vi "读写字节数组DEMO.vi"() -> ()   [LabVIEW 2012]
panel:
  out "Receive":dbl(graph)
  out "Send":dbl(graph)
  in  "停止":bool
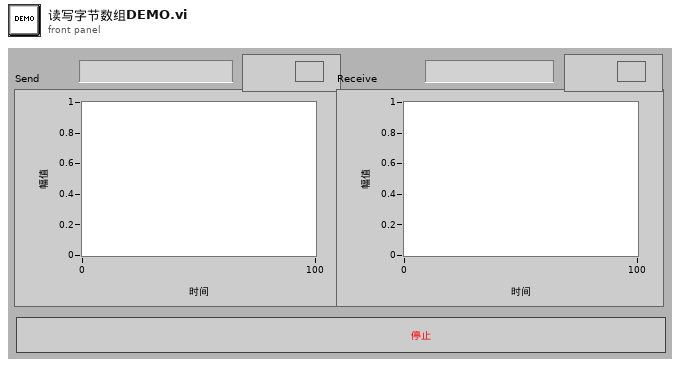
[diagram p1: front panel]
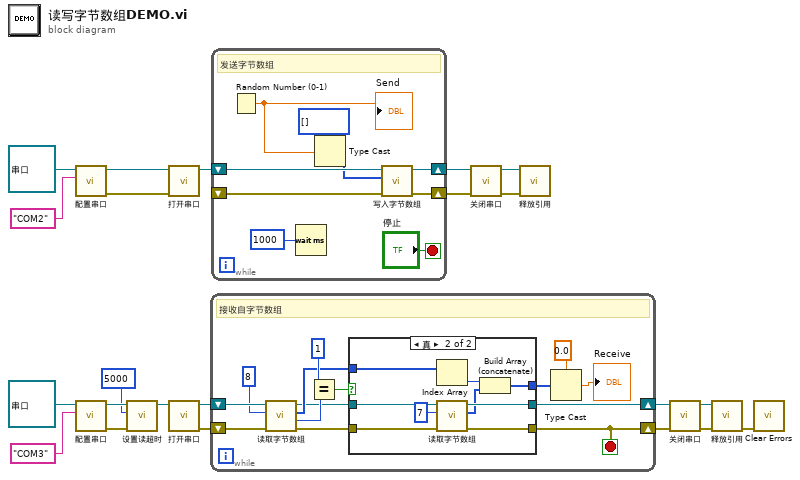
[diagram p0: block diagram]
diagram:
  n1 = call "配置串口.vi"("Port Name"="COM2", "COM 输入"=refnum<class "串口.lvclass"> refnum ("串口.lvclass")) -> ("error out"=w19:errorcluster, "COM 输出"=w20:refnum<class "串口.lvclass">)  [unwired: 8 in]
  n2 = call "配置串口.vi"("Port Name"="COM3", "COM 输入"=refnum<class "串口.lvclass"> refnum ("串口.lvclass")) -> ("error out"=w3:errorcluster, "COM 输出"=w4:refnum<class "串口.lvclass">)  [unwired: 8 in]
  n3 = call "设置读超时.vi"("error in (no error)"=w3, "ReadTimeout"=5000, "串口 输入"=w4) -> ("串口 输出"=w1:refnum<class "串口.lvclass">)  [unwired: 7 in, 1 out]
  n4 = call "打开串口.vi"("error in (no error)"=w19, "串口 输入"=w20) -> ("串口 输出"=w18:refnum<class "串口.lvclass">)  [unwired: 8 in, 1 out]
  n5 = call "打开串口.vi"("串口 输入"=w1) -> ("error out"=w8:errorcluster, "串口 输出"=w9:refnum<class "串口.lvclass">)  [unwired: 9 in]
  n6 = while {
    shift-right: [w23] -> w7
    shift-left: w8 -> [w35]
    shift-right: [w27] -> w6
    shift-left: w9 -> [w36]
    stop <- w23 stop-if-true
    # "接收自字节数组"
    n7 = call "读取字节数组.vi"("error in (no error)"=w35, "count"=8, "串口 输入"=w36) -> ("error out"=w29:errorcluster, "Read"=w33:i32, "Bytes"=w31:u8[], "串口 输出"=w28:refnum<class "串口.lvclass">)  [unwired: 5 in]
    n8 = Equal?(x=1 ("y"), y=w33) -> (x = y?=w30:bool)
    n9 = case shown="真" w30 {
      tunnel: w31 -> [w39 w43]
      tunnel: [w39 w40] -> w26
      tunnel: w29 -> [w37 w48]
      tunnel: [w37 w47] -> w23
      tunnel: w28 -> [w38 w46]
      tunnel: [w38 w44] -> w27
      frame False {
      }
      frame True {
        n10 = Index Array(array=w43) -> (element=w42:u8)  [unwired: 1 in]
        n11 = call "读取字节数组.vi"("error in (no error)"=w48, "count"=7, "串口 输入"=w46) -> ("error out"=w47:errorcluster, "Bytes"=w41:u8[], "串口 输出"=w44:refnum<class "串口.lvclass">)  [unwired: 5 in, 1 out]
        n12 = Build Array (concatenate)(w42, w41) -> (w40:u8[])
      }
    }
    n13 = Type Cast(type=0.0, x=w26) -> (*(type *) &x=→"Receive":dbl)
  }
  n14 = while "While循环" {
    shift-right: [w52] -> w16
    shift-left: _ -> [w54]
    shift-right: [w53] -> w17
    shift-left: w18 -> [w55]
    stop <- "停止" stop-if-true
    # "发送字节数组"
    n15 = Random Number (0-1)() -> (number: 0 to 1=w49:dbl)
    "Send" <- w49
    n16 = Wait (ms)(milliseconds to wait=u32 1000 ("等待时间（毫秒）")) -> ()  [unwired: 1 out]
    n17 = Type Cast(type=u8[] [], x=w49) -> (*(type *) &x=w50:u8[])
    n18 = call "写入字节数组.vi"("error in (no error)"=w54, "Bytes"=w50, "串口 输入"=w55) -> ("error out"=w52:errorcluster, "串口 输出"=w53:refnum<class "串口.lvclass">)  [unwired: 7 in]
  }
  n19 = call "关闭串口.vi"("error in (no error)"=w16, "串口 输入"=w17) -> ("error out"=w15:errorcluster, "串口 输出"=w14:refnum<class "串口.lvclass">)  [unwired: 8 in]
  n20 = call "释放引用.vi"("error in (no error)"=w15, "串口 输入"=w14) -> ()  [unwired: 8 in, 2 out]
  n21 = call "关闭串口.vi"("error in (no error)"=w7, "串口 输入"=w6) -> ("error out"=w10:errorcluster, "串口 输出"=w11:refnum<class "串口.lvclass">)  [unwired: 8 in]
  n22 = call "释放引用.vi"("error in (no error)"=w10, "串口 输入"=w11) -> ("error out"=w5:errorcluster)  [unwired: 8 in, 1 out]
  n23 = call <vilib>:"Clear Errors.vi"("error in (no error)"=w5) -> ()  [unwired: 6 in, 1 out]
